vi "g_setting.vi"() -> ()   [LabVIEW 2015, in "Admin_Actor.lvlib"]
uses:
  Admin_Actor.lvlib
panel:
  in  "Time Stamp":timestamp=timestamp(3558323554.214689 s since 1904-01-01) format="%<%x>T"
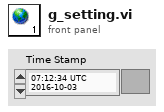
[diagram p1: front panel]
diagram:
